vi "Read Group.vi"(8 "error in (no error)":errorcluster, 11 "Async Message in":refnum<class "Async Message.lvclass">) -> (0 "error out":errorcluster, 2 "Group":u16 format="%04x", 3 "Async Message out":refnum<class "Async Message.lvclass">)   [LabVIEW 2016]
uses:
  Async Message.lvclass
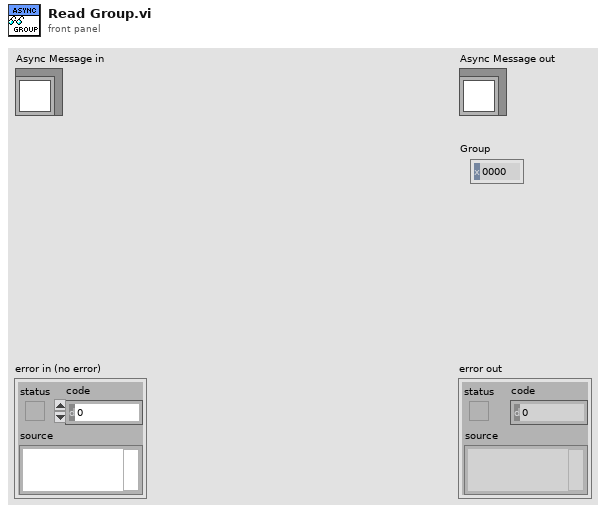
[diagram p1: front panel]
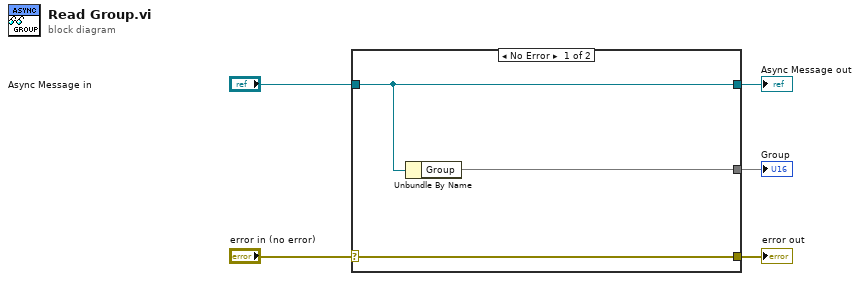
[diagram p0: block diagram]
diagram:
  n1 = case shown="No Error" "error in (no error)" {
    selector: "error in (no error)" -> [w8 w9]
    tunnel: [w8 w9] -> w4
    tunnel: [w7 w10] -> w2
    tunnel: "Async Message in" -> [w7 w10]
    tunnel: [w6 _] -> w1
    frame No Error {
      n2 = Unbundle By Name(w7) -> ("Group"=w6)
    }
    frame Error {
    }
  }
  "error out" <- w4
  "Async Message out" <- w2
  "Group" <- w1
